vi "WebVGA main demo.vi"() -> ()   [LabVIEW 2014]
uses:
  Global vars.vi
panel:
  in  "stop":bool
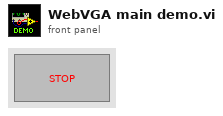
[diagram p1: front panel]
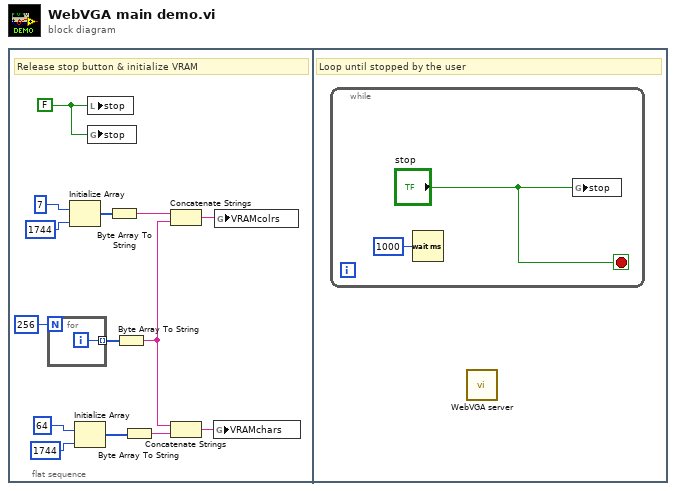
[diagram p0: block diagram]
diagram:
  n1 = flat-sequence {
    frame #0 {
      w14 = FALSE ("stop")
      # "Release stop button & initialize VRAM"
      n2 = for {
        N: 256 -> [_]
        tunnel: [w15] -> w6 mode=indexing
        i -> [w15]
      }
      n3 = Initialize Array(u8 7 ("element"), 1744 ("dimension size")) -> (w10:u8[])
      n4 = Initialize Array(u8 64 ("element"), 1744 ("dimension size")) -> (w11:u8[])
      n5 = local write "stop"(w14) -> ()
      n6 = global write "Global vars.vi" "stop"(w14) -> ()
      n7 = Byte Array To String(unsigned byte array=w10) -> (string=w5:string)
      n8 = Byte Array To String(unsigned byte array=w6) -> (string=w1:string)
      n9 = Byte Array To String(unsigned byte array=w11) -> (string=w2:string)
      n10 = Concatenate Strings(w5, w1) -> (w4:string)
      n11 = Concatenate Strings(w1, w2) -> (w3:string)
      n12 = global write "Global vars.vi" "VRAMchars"(w3) -> ()
      n13 = global write "Global vars.vi" "VRAMcolrs"(w4) -> ()
    }
    frame #1 {
      # "Loop until stopped by the user"
      n14 = while {
        stop <- "stop" stop-if-true
        n15 = Wait (ms)(milliseconds to wait=u32 1000) -> ()  [unwired: 1 out]
        n16 = global write "Global vars.vi" "stop"("stop") -> ()
      }
      n17 = call "WebVGA server.vi"() -> ()  [unwired: 10 in, 2 out]
    }
  }
